vi "생산자소비자(이벤트).vi"() -> ()   [LabVIEW 2014]
uses:
  <vilib>/Analysis/NI_AALBase.lvlib
panel:
  in  "기다림":i32
  out "웨이브폼 그래프":dbl[](graph)
  in  "정지":bool
  in  "확인 버튼":bool
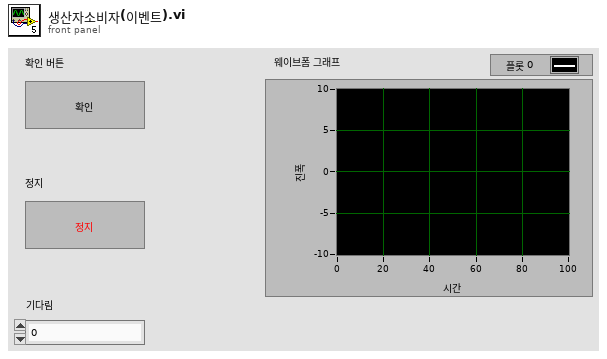
[diagram p1: front panel]
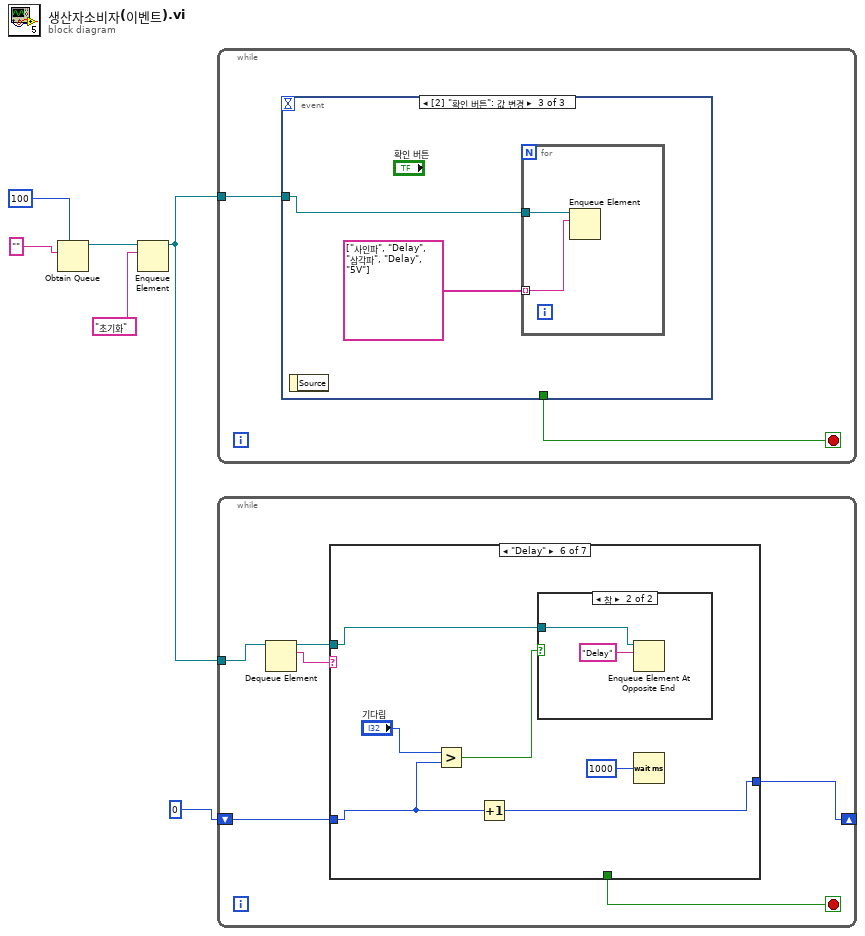
[diagram p0: block diagram]
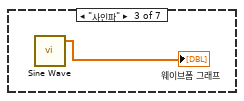
[diagram p4: hidden frame]
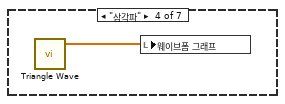
[diagram p5: hidden frame]
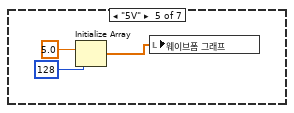
[diagram p6: hidden frame]
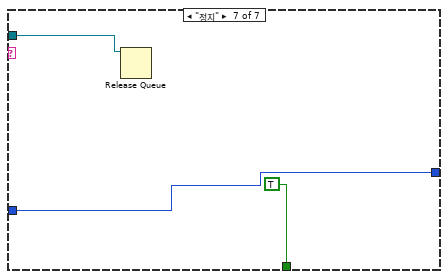
[diagram p8: hidden frame]
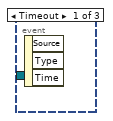
[diagram p9: hidden frame]
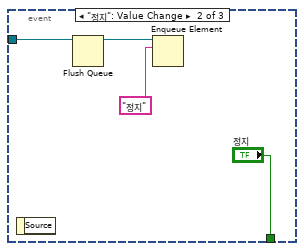
[diagram p10: hidden frame]
diagram:
  n1 = Obtain Queue(max queue size (-1, unlimited)=100 ("최대 큐 크기(-1,제한없음)"), element data type="") -> (queue out=w6:refnum<queue>)  [unwired: 3 in, 2 out]
  n2 = Enqueue Element(queue=w6, element="초기화" ("원소")) -> (queue out=w2:refnum<queue>)  [unwired: 2 in, 2 out]
  n3 = while {
    tunnel: w2 -> [w7]
    stop <- w8 stop-if-true
    n4 = event shown="[2] \"확인 버튼\": 값 변경" {
      selector: _ -> [_ _ _]
      dyn-events: _ -> [_ _ _]
      timeout: _ -> [_ _ _]
      tunnel: [_ "정지" _] -> w8
      tunnel: w7 -> [_ w9 w14]
      event Timeout {
        n5 = event-data() -> ()  [unwired: 1 in, 3 out]
      }
      event "정지": Value Change {
        n6 = event-data() -> ()  [unwired: 1 in, 1 out]
        n7 = Flush Queue(queue=w9) -> (queue out=w11:refnum<queue>)  [unwired: 1 in, 2 out]
        n8 = Enqueue Element(queue=w11, element="정지" ("원소")) -> ()  [unwired: 2 in, 3 out]
      }
      event "확인 버튼": Value Change {
        n9 = event-data() -> ()  [unwired: 1 in, 1 out]
        n10 = for {
          tunnel: w14 -> [w16]
          tunnel: string[] ["사인파", "Delay", "삼각파", "Delay", "5V"] -> [w15] mode=indexing
          n11 = Enqueue Element(queue=w16, element=w15) -> ()  [unwired: 2 in, 3 out]
        }
      }
    }
  }
  n12 = while {
    tunnel: w2 -> [w22]
    shift-right: [w19] -> _
    shift-left: 0 -> [w18]
    stop <- w20 stop-if-true
    n13 = Dequeue Element(queue=w22) -> (queue out=w17:refnum<queue>, element=w21:string)  [unwired: 2 in, 2 out]
    n14 = case shown="\"Delay\"" w21 {
      tunnel: [_ _ _ _ _ _ TRUE] -> w20
      tunnel: [_ _ _ _ _ w33 w37] -> w19
      tunnel: w18 -> [_ _ _ _ _ w32 w37]
      tunnel: w17 -> [_ _ _ _ _ w29 w36]
      frame Default {
      }
      frame "초기화" {
      }
      frame "사인파" {
        n15 = call <vilib>:"Sine Wave.vi"() -> ("sine wave"=→"웨이브폼 그래프":dbl[])  [unwired: 5 in, 2 out]
      }
      frame "삼각파" {
        n16 = call <vilib>:"Triangle Wave.vi"() -> ("triangle wave"=w24:dbl[])  [unwired: 5 in, 2 out]
        n17 = local write "웨이브폼 그래프"(w24) -> ()
      }
      frame "5V" {
        n18 = Initialize Array(5.0 ("원소"), 128 ("차원 크기")) -> (w25:dbl[])
        n19 = local write "웨이브폼 그래프"(w25) -> ()
      }
      frame "Delay" {
        n20 = Greater?(x="기다림", y=w32) -> (0:w30:bool)
        n21 = Increment(x=w32) -> (x+1=w33:i32)
        n22 = case shown="참" w30 {
          tunnel: w29 -> [_ w35]
          frame False {
          }
          frame True {
            n23 = Enqueue Element At Opposite End(queue=w35, element="Delay" ("원소")) -> ()  [unwired: 2 in, 3 out]
          }
        }
        n24 = Wait (ms)(milliseconds to wait=u32 1000 ("대기 시간(ms)")) -> ()  [unwired: 1 out]
      }
      frame "정지" {
        n25 = Release Queue(queue=w36) -> ()  [unwired: 2 in, 3 out]
      }
    }
  }
